vi "Get Ctls Ref By Class Name.vi"(8 "error in (no error)":errorcluster, 10 "Control Class":string(combo), 11 "Abstruct View in":refnum<class "Abstruct View.lvclass">) -> (0 "error out":errorcluster, 2 "refs":refnum<vi>[](array[refnum]), 3 "Abstruct View out":refnum<class "Abstruct View.lvclass">)   [LabVIEW 2020, in "Abstruct View.lvlib" / "Abstruct View.lvclass"]
uses:
  Abstruct View.lvclass
  Abstruct View.lvclass/Abstruct View.ctl
  Data Accessors/Read Core VI.vi
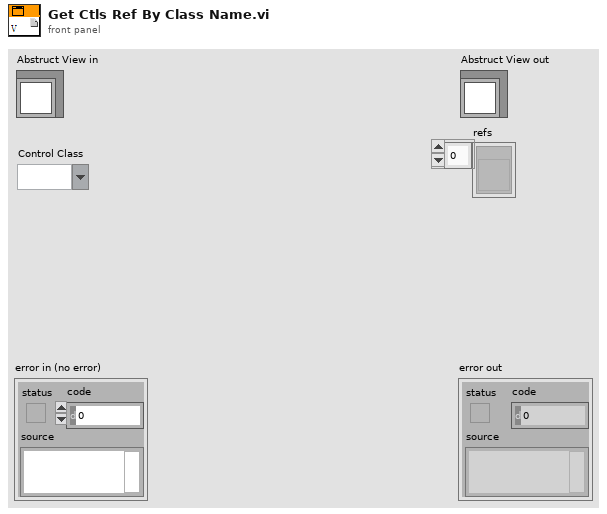
[diagram p1: front panel]
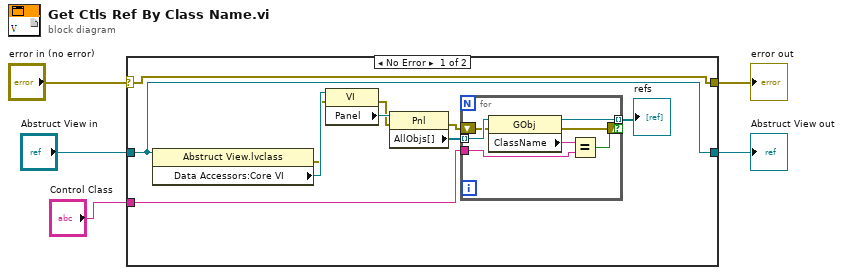
[diagram p0: block diagram]
diagram:
  n1 = case shown="No Error" "error in (no error)" {
    selector: "error in (no error)" -> [w15 w24]
    tunnel: [w15 w24] -> w4
    tunnel: [w11 w23] -> w2
    tunnel: "Abstruct View in" -> [w11 w23]
    tunnel: "Control Class" -> [w6 _]
    frame No Error {
      n2 = property class="Abstruct View.lvclass"(reference=w11) -> (error out=w9:errorcluster, "Data Accessors:Core VI"=w10:refnum<vi>)  [unwired: 1 in, 1 out]
      n3 = property class="VI"(reference=w10, error in=w9) -> (error out=w8:errorcluster, "Panel"=w14:refnum<vi>)  [unwired: 1 out]
      n4 = property class="Pnl"(reference=w14, error in=w8) -> (error out=w7:errorcluster, "AllObjs[]"=w13:refnum<vi>[])  [unwired: 1 out]
      n5 = for {
        tunnel: w13 -> [w22] mode=indexing
        tunnel: [w20] -> w12 mode=indexing if=w19
        tunnel: w6 -> [w18]
        shift-right: [w16] -> _
        shift-left: w7 -> [w17]
        n6 = property class="GObj"(reference=w22, error in=w17) -> (reference out=w20:refnum<vi>, error out=w16:errorcluster, "ClassName"=w21:string)
        n7 = Equal?(x=w21, y=w18) -> (x = y?=w19:bool)
      }
      "refs" <- w12
    }
    frame Error {
    }
  }
  "error out" <- w4
  "Abstruct View out" <- w2
